vi "signal_generator.vi"() -> ()   [LabVIEW 2015]
uses:
  <vilib>/DAQmx/write.llb/DAQmx Write (Analog 1D DBL 1Chan NSamp).vi
  <vilib>/DAQmx/create/channels.llb/DAQmx Create Channel (AO-Voltage-Basic).vi
  <vilib>/DAQmx/configure/timing.llb/DAQmx Timing (Sample Clock).vi
  <vilib>/DAQmx/miscellaneous.llb/DAQmx Fill In Error Info.vi
  <vilib>/measure/NI_MABase.lvlib
panel:
  in  "sync output channel":tag
  in  "sine amplitude":dbl=1.0 format="%#_13g"
  in  "square amplitude":dbl=9.0 format="%#_13g"
  in  "Analog Output Channel":tag
  in  "sampling info":cluster{"Fs":dbl, "#s":dbl}={"Fs"=5000.0, "#s"=1000.0} {"Fs" format="%.2p"}
  in  "square frequency":dbl=0.0078125 format="%0.4e"
  in  "sine frequency":dbl=0.0078125 format="%0.4e"
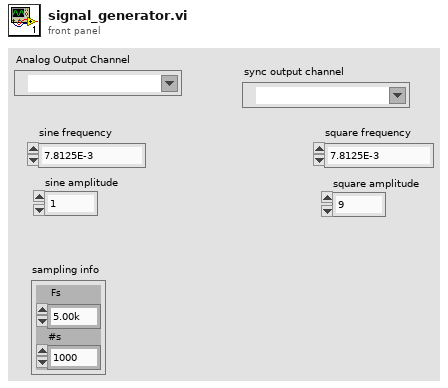
[diagram p1: front panel]
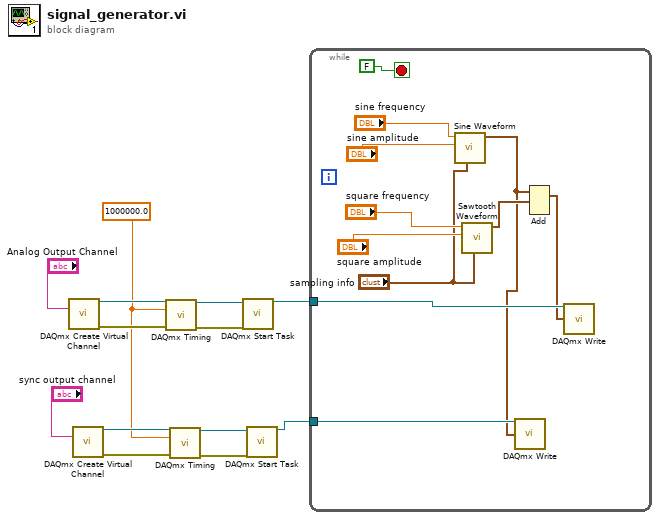
[diagram p0: block diagram]
diagram:
  w2 = 1000000.0 ("rate")
  n1 = call-poly <vilib>:"DAQmx Create Virtual Channel.vi"("physical channels"="Analog Output Channel") -> ("task out"=w11:refnum<k21>, "error out"=w13:errorcluster)  [unwired: 8 in, 5 out]
  n2 = call-poly <vilib>:"DAQmx Create Virtual Channel.vi"("physical channels"="sync output channel") -> ("task out"=w5:refnum<k21>, "error out"=w7:errorcluster)  [unwired: 8 in, 5 out]
  n3 = call-poly <vilib>:"DAQmx Timing.vi"("task/channels in"=w11, "rate"=w2, "error in"=w13) -> ("task out"=w10:refnum<k21>, "error out"=w12:errorcluster)  [unwired: 4 in, 7 out]
  n4 = call-poly <vilib>:"DAQmx Timing.vi"("task/channels in"=w5, "rate"=w2, "error in"=w7) -> ("task out"=w4:refnum<k21>, "error out"=w6:errorcluster)  [unwired: 4 in, 7 out]
  n5 = call <vilib>:"DAQmx Start Task.vi"("task/channels in"=w10, "error in"=w12) -> ("task out"=w8:refnum<k21>)  [unwired: 13 out]
  n6 = call <vilib>:"DAQmx Start Task.vi"("task/channels in"=w4, "error in"=w6) -> ("task out"=w1:refnum<k21>)  [unwired: 13 out]
  n7 = while {
    tunnel: w8 -> [w17]
    tunnel: w1 -> [w15]
    stop <- FALSE stop-if-true
    n8 = call <vilib>:"Sine Waveform.vi"("sampling info"="sampling info", "amplitude"="sine amplitude", "frequency"="sine frequency") -> ("signal out"=w14:waveform(dbl))  [unwired: 7 in, 1 out]
    n9 = call <vilib>:"Sawtooth Waveform.vi"("sampling info"="sampling info", "amplitude"="square amplitude", "frequency"="square frequency") -> ("signal out"=w22:waveform(dbl))  [unwired: 7 in, 1 out]
    n10 = call-poly <vilib>:"DAQmx Write.vi"("task/channels in"=w15, "data"=w14) -> ()  [unwired: 2 in, 12 out]
    n11 = Add(1:w22, 2:w14) -> (0:w16:waveform(dbl))  [unwired: 1 in, 1 out]
    n12 = call-poly <vilib>:"DAQmx Write.vi"("task/channels in"=w17, "data"=w16) -> ()  [unwired: 2 in, 12 out]
  }
